vi "Get UI Ref.vi"(8 "error in (no error)":errorcluster, 11 "9401 in":refnum<class "9401.lvclass">) -> (0 "error out":errorcluster, 1 "Show SubPanel?":bool, 2 "VI Refnum":refnum<vi>, 3 "9401 out":refnum<class "9401.lvclass">)   [LabVIEW 2011, in "Modules.lvlib" / "9401.lvclass"]
uses:
  9401.lvclass
  SD Module/SD Module.lvclass
  RSI Module/RSI Module.lvclass
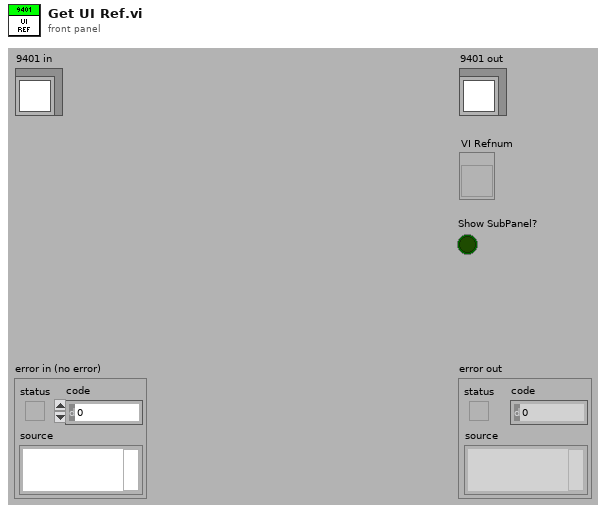
[diagram p1: front panel]
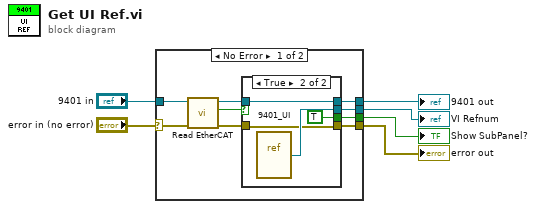
[diagram p0: block diagram]
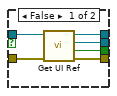
[diagram p2: hidden frame]
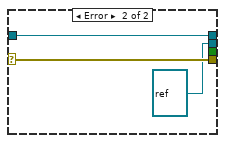
[diagram p3: hidden frame]
diagram:
  n1 = case shown="No Error" "error in (no error)" {
    selector: "error in (no error)" -> [w12 w28]
    tunnel: [w7 w28] -> w3
    tunnel: [w9 w27] -> w5
    tunnel: "9401 in" -> [w13 w27]
    tunnel: [w15 refnum<vi> refnum] -> w2
    tunnel: [w14 _] -> w1
    frame No Error {
      n2 = call "Read EtherCAT.vi"("error in (no error)"=w12, "RSI Module in"=w13) -> ("error out"=w8:errorcluster, "EtherCAT?"=w11:bool, "RSI Module out"=w10:refnum<class "9401.lvclass">)  [unwired: 7 in]
      n3 = case shown="True" w11 {
        tunnel: [w21 w25] -> w15
        tunnel: [w20 TRUE] -> w14
        tunnel: w10 -> [w19 w22]
        tunnel: [w18 w22] -> w9
        tunnel: w8 -> [w17 w23]
        tunnel: [w16 w23] -> w7
        frame False {
          n4 = call-parent "Get UI Ref.vi"("error in (no error)"=w17, "SD Module in"=w19) -> ("error out"=w16:errorcluster, "Show SubPanel?"=w20:bool, "VI Refnum"=w21:refnum<vi>, "SD Module out"=w18:refnum<class "9401.lvclass">)  [unwired: 6 in]
        }
        frame True {
          n5 = vi-ref "9401_UI.vi"() -> (w25:refnum<vi>)
        }
      }
    }
    frame Error {
    }
  }
  "error out" <- w3
  "9401 out" <- w5
  "VI Refnum" <- w2
  "Show SubPanel?" <- w1
